vi "CRYCursor Move.vi"(9 "x":i16, 10 "Active Cursor":u32, 11 "Graph Ref":refnum<vi>) -> ()   [LabVIEW 2013]
panel:
  out "current":dbl
  out "before":dbl
  out "after":dbl
  out "total":i32
  out "current index":i32
  out "same index":i32
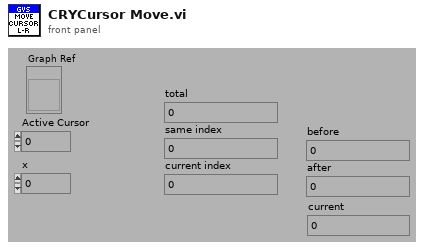
[diagram p1: front panel]
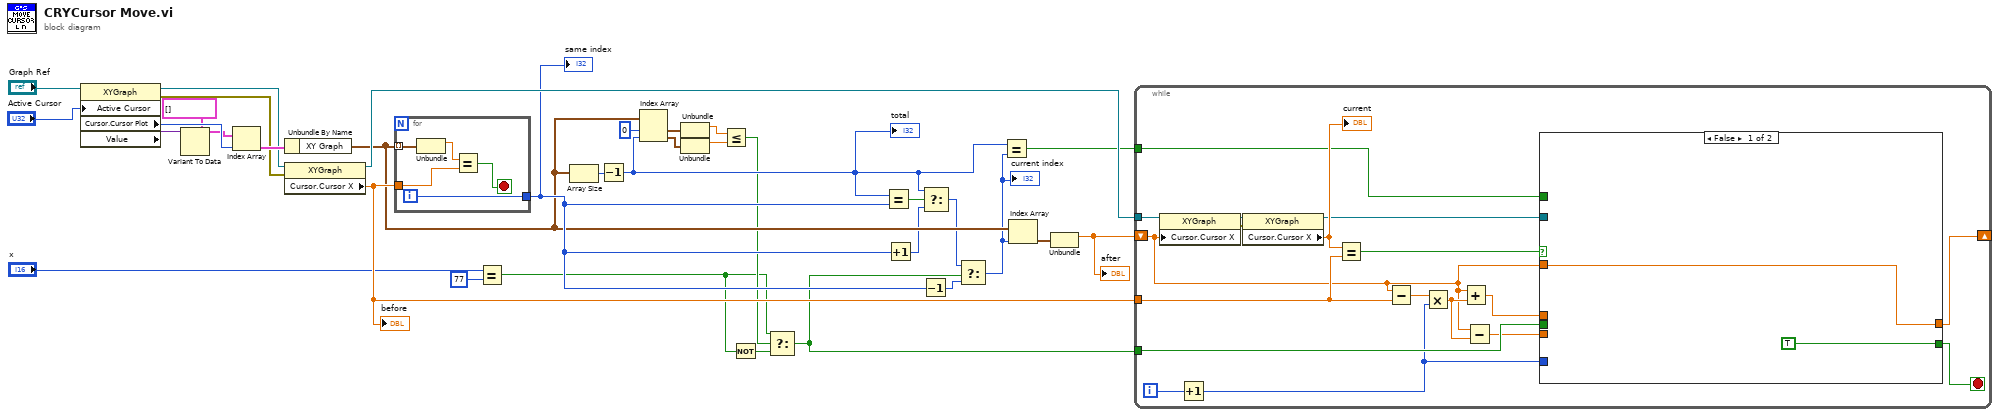
[diagram p0: block diagram]
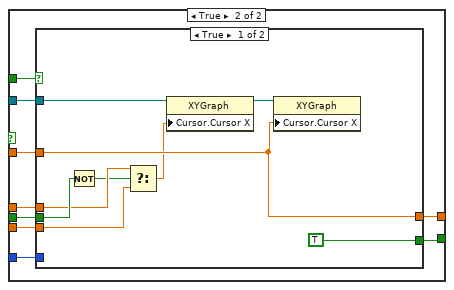
[diagram p2: hidden frame]
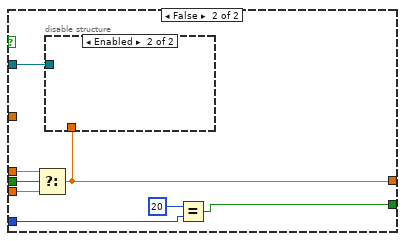
[diagram p3: hidden frame]
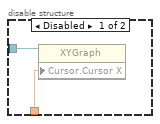
[diagram p4: hidden frame]
diagram:
  n1 = property on="Property Node" class="XYGraph"(reference="Graph Ref", "Active Cursor"="Active Cursor") -> (reference out=w30:refnum<vi>, error out=w32:errorcluster, "Cursor.Cursor Plot"=w34:i32, "Value"=w27:variant)  [unwired: 1 in]
  n2 = Variant To Data(type=cluster{"XY Graph":cluster{dbl, dbl}[]}[] [] ("XY Graph"), Variant=w27) -> (data=w25:cluster{"XY Graph":cluster{dbl, dbl}[]}[])  [unwired: 1 in, 1 out]
  n3 = Index Array(array=w25, index=w34) -> (element=w33:cluster{"XY Graph":cluster{dbl, dbl}[]})
  n4 = Unbundle By Name(w33) -> ("XY Graph"=w19:cluster{dbl, dbl}[])
  n5 = property on="Property Node" class="XYGraph"(reference=w30, error in=w32) -> (reference out=w29:refnum<vi>, "Cursor.Cursor X"=w22:dbl)  [unwired: 1 out]
  "before" <- w22
  n6 = for {
    tunnel: w19 -> [w39] mode=indexing
    tunnel: w22 -> [w37]
    tunnel: [w36] -> w20
    i -> [w36]
    stop <- w35 stop-if-true
    n7 = Unbundle(w39) -> (w38:dbl)  [unwired: 1 out]
    n8 = Equal?(x=w38, y=w37) -> (x = y?=w35:bool)
  }
  "same index" <- w20
  n9 = Equal?(x="x", y=i16 77) -> (x = y?=w3:bool)
  n10 = Array Size(array=w19) -> (size(s)=w23:i32)
  n11 = Decrement(x=w23) -> (x-1=w18:i32)
  "total" <- w18
  n12 = Index Array(array=w19, index #1=0 ("index"), index #2=w18) -> (element #1=w16:cluster{dbl, dbl}, element #2=w15:cluster{dbl, dbl})
  n13 = Unbundle(w16) -> (w14:dbl)  [unwired: 1 out]
  n14 = Unbundle(w15) -> (w13:dbl)  [unwired: 1 out]
  n15 = Less Or Equal?(x=w14, y=w13) -> (x <= y?=w4:bool)
  n16 = Not(x=w3) -> (.not. x?=w2:bool)
  n17 = Select(t=w3, s=w4, f=w2) -> (s? t:f=w1:bool)
  n18 = Equal?(x=w18, y=w20) -> (x = y?=w10:bool)
  n19 = Increment(x=w20) -> (x+1=w9:i32)
  n20 = Decrement(x=w20) -> (x-1=w11:i32)
  n21 = Select(t=w18, s=w10, f=w9) -> (s? t:f=w8:i32)
  n22 = Select(t=w8, s=w1, f=w11) -> (s? t:f=w5:i32)
  "current index" <- w5
  n23 = Equal?(x=w18, y=w5) -> (x = y?=w7:bool)
  n24 = Index Array(array=w19, index=w5) -> (element=w12:cluster{dbl, dbl})
  n25 = Unbundle(w12) -> (w6:dbl)  [unwired: 1 out]
  "after" <- w6
  n26 = while {
    tunnel: w29 -> [w57]
    tunnel: w22 -> [w52]
    tunnel: w1 -> [w51]
    tunnel: w7 -> [w46]
    shift-right: [w42] -> _
    shift-left: w6 -> [w45]
    i -> [w44]
    stop <- w41 stop-if-true
    n27 = property on="Property Node" class="XYGraph"(reference=w57, "Cursor.Cursor X"=w45) -> (reference out=w56:refnum<vi>, error out=w55:errorcluster)  [unwired: 1 in]
    n28 = Increment(x=w44) -> (x+1=w40:i32)
    n29 = property on="Property Node" class="XYGraph"(reference=w56, error in=w55) -> (reference out=w53:refnum<vi>, "Cursor.Cursor X"=w54:dbl)  [unwired: 1 out]
    "current" <- w54
    n30 = Equal?(x=w54, y=w52) -> (x = y?=w43:bool)
    n31 = Subtract(x=w45, y=w52) -> (x-y=w47:dbl)
    n32 = Multiply(x=w47, y=w40) -> (x*y=w50:dbl)
    n33 = Add(x=w45, y=w50) -> (x+y=w48:dbl)
    n34 = Subtract(x=w45, y=w50) -> (x-y=w49:dbl)
    n35 = case shown="False" w43 {
      tunnel: w53 -> [_ w68]
      tunnel: w51 -> [_ w67]
      tunnel: w49 -> [_ w65]
      tunnel: w48 -> [_ w66]
      tunnel: w46 -> [_ w64]
      tunnel: w45 -> [w59 w63]
      tunnel: [w59 w62] -> w42
      tunnel: [TRUE w61] -> w41
      tunnel: w40 -> [_ w60]
      frame False {
      }
      frame True {
        n36 = case shown="True" w64 {
          tunnel: w68 -> [w77 w85]
          tunnel: w67 -> [w76 w84]
          tunnel: w66 -> [w75 w83]
          tunnel: w65 -> [w74 w82]
          tunnel: w63 -> [w73 _]
          tunnel: [w73 w81] -> w62
          tunnel: [TRUE w78] -> w61
          tunnel: w60 -> [_ w80]
          frame True {
            n37 = Not(x=w76) -> (.not. x?=w70:bool)
            n38 = Select(t=w75, s=w70, f=w74) -> (s? t:f=w69:dbl)
            n39 = property on="Property Node" class="XYGraph"(reference=w77, "Cursor.Cursor X"=w69) -> (reference out=w71:refnum<vi>)  [unwired: 1 in, 1 out]
            n40 = property on="Property Node" class="XYGraph"(reference=w71, "Cursor.Cursor X"=w73) -> ()  [unwired: 1 in, 2 out]
          }
          frame False {
            n41 = Select(t=w83, s=w84, f=w82) -> (s? t:f=w81:dbl)
            n42 = disable-structure shown="Enabled" {
              disable-tunnel: w85 -> [w87 _]
              disable-tunnel: w81 -> [w86 _]
              frame Disabled {
                n43 = property on="Property Node" class="XYGraph"(reference=w87, "Cursor.Cursor X"=w86) -> ()  [unwired: 1 in, 2 out]
              }
              frame Enabled {
              }
            }
            n44 = Equal?(x=20, y=w80) -> (x = y?=w78:bool)
          }
        }
      }
    }
  }
